vi "Get Configuration Default.vi"(8 "error in (no error)":errorcluster) -> (0 "error out":errorcluster, 3 "Measurement Configuration Default":T1={"Load Current in A"=0.005, "Nominal Output Voltage in V"=3.3, "Start"=4.0, "Stop"=6.0, "Step"=0.1, "Input SMU"="", "Load SMU"="", "Input DMM"="", "Load DMM"=""} {"Nominal Output Voltage in V" format="%#_13g"; "Load Current in A" format="%#_13g"})   [LabVIEW 2020, in "LineRegulation.lvlib"]
uses:
  LineRegulation.lvlib
  Measurement Configuration.ctl
  e54118e4-a0f5-41b8-bd23-fc2d3fb72aa9.vi
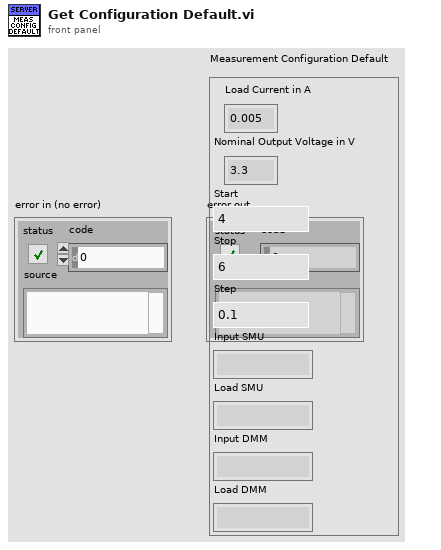
[diagram p1: front panel]
types:
  T1 = typedef "LineRegulation.lvlib/Measurement Configuration.ctl" = cluster{"Load Current in A":dbl, "Nominal Output Voltage in V":dbl, "Start":dbl, "Stop":dbl, "Step":dbl, "Input SMU":string, "Load SMU":string, "Input DMM":string, "Load DMM":string}
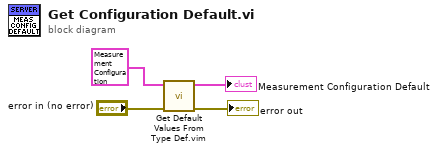
[diagram p0: block diagram]
diagram:
  n1 = call "Get Default Values From Type Def.vim"("error in (no error)"="error in (no error)", "Type Def"=T1 {"Load Current in A"=0.005, "Nominal Output Voltage in V"=3.3, "Start"=4.0, "Stop"=6.0, "Step"=0.1, "Input SMU"="", "Load SMU"="", "Input DMM"="", "Load DMM"=""} ("Measurement Configuration")) -> ("error out"=→"error out":errorcluster, "Default Values"=→"Measurement Configuration Default":T1)  [unwired: 8 in]
